vi "Semaphore Timed Wait (relative seconds).vi"(8 "error in (no error)":errorcluster, 10 "relative timeout (seconds)":dbl, 11 "Semaphore in":T1) -> (0 "error out":errorcluster, 2 "timed out?":bool, 3 "Semaphore out":T1)   [LabVIEW 2016, in "Linux RT IPC.POSIX Threads.lvlib" / "Semaphore.lvclass"]
doc: "Calls sem_timedwait() on the semaphore object encapsulated by Semaphore.\n\nThis VI attempts to decrement the value of the semaphore by 1 within a timeout period. If the semaphore can be decremented within the timeout period, this VI returns indicating it was successful. Otherwise, this VI returns indicating the semaphore was never set.\n\nRefer to online POSIX documentation for more information."
uses:
  Semaphore.lvclass
  Controls/reference.ctl
  C:/Git/SourceTree/LinuxRT-IPC/Source/POSIX Threads/Classes/POSIX Thread Object/POSIX Thread Object.lvclass
  <vilib>/NI/NI Linux RT Utilities/Controls/Public/C Enums/clockid_t.ctl
  POSIX Thread Object/POSIX Thread Object.lvclass/POSIX Thread Object.ctl
  POSIX Thread Object/Private VIs/libpthread path.vi
  <vilib>/NI/NI Linux RT Utilities/VIs/Public/Convert Types/convert timespec 64 to timespec 32.vi
  POSIX Thread Object/Private VIs/get pthread error.vi
  <vilib>/NI/NI Linux RT Errno/VIs/Public/SubVIs/errno enum to number.vi
  <vilib>/NI/NI Linux RT Errno/VIs/Public/Get Errno Value for Calling Thread.vi
  <vilib>/NI/NI Linux RT Utilities/VIs/Public/Time/Increment Time (timespec).vi
  <vilib>/NI/NI Linux RT Utilities/VIs/Public/Time/Get Clock Time (timespec).vi
  POSIX Thread Object/POSIX Thread Object.lvclass
  <vilib>/NI/NI Linux RT Utilities/Linux RT Utilities.lvlib
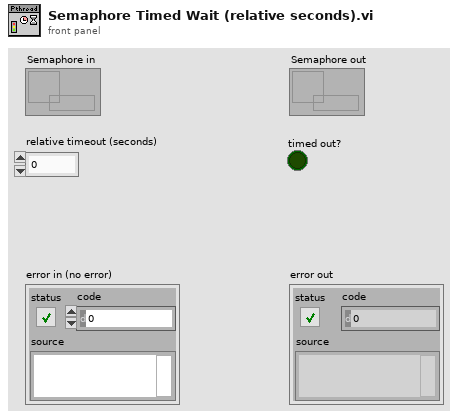
[diagram p1: front panel]
types:
  T1 = typedef "Linux RT IPC.POSIX Threads.lvlib/Semaphore.lvclass/reference.ctl" = refnum<data-value>
  T2 = typedef "Linux RT Utilities.lvlib/clockid_t.ctl" = enum16{"Realtime", "Monotonic"}
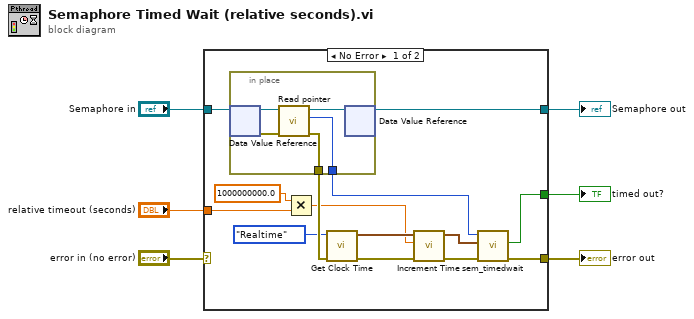
[diagram p0: block diagram]
diagram:
  n1 = case shown="No Error" "error in (no error)" {
    selector: "error in (no error)" -> [_ w26]
    tunnel: "Semaphore in" -> [w20 w27]
    tunnel: [w19 w27] -> w3
    tunnel: [w18 w26] -> w4
    tunnel: "relative timeout (seconds)" -> [w8 _]
    tunnel: [w17 _] -> w1
    frame No Error {
      n2 = in-place {
        in-place-border: [w22] -> w15
        in-place-border: [w21] -> w16
        n3 = in-place-dvr #1(w20) -> (w25:refnum<class "Semaphore.lvclass">, w24:errorcluster)
        n4 = call "Read pointer.vi"("error in (no error)"=w24, "POSIX Thread Object in"=w25) -> ("error out"=w22:errorcluster, "pointer"=w21:u64, "POSIX Thread Object out"=w23:refnum<class "Semaphore.lvclass">)  [unwired: 7 in]
        n5 = in-place-dvr #1(w23) -> (w19:T1)  [unwired: 1 out]
      }
      n6 = Multiply(x=1000000000.0, y=w8) -> (x*y=w7:dbl)
      n7 = call-poly <vilib>:"Get Clock Time.vi"("error in (no error)"=w15, "clock id (realtime)"=clockid_t."Realtime" ("clock id (monotonic)")) -> ("error out"=w13:errorcluster, "timespec"=w12:cluster{"sec":u64, "nsec":u64})  [unwired: 8 in]
      n8 = call-poly <vilib>:"Increment Time.vi"("error in (no error)"=w13, "nanos offset"=w7, "timespec in"=w12) -> ("error out"=w10:errorcluster, "timespec out"=w11:cluster{"sec":u64, "nsec":u64})  [unwired: 7 in]
      n9 = call "sem_timedwait.vi"("error in (no error)"=w10, "absolute timeout"=w11, "sempahore ptr in"=w16) -> ("error out"=w18:errorcluster, "timed out?"=w17:bool)  [unwired: 6 in, 1 out]
    }
    frame Error {
    }
  }
  "error out" <- w4
  "Semaphore out" <- w3
  "timed out?" <- w1
